vi "Main.vi"(8 "error in":errorcluster, 11 "DataSave Worker in":refnum<class "DataSave Worker.lvclass">) -> (0 "error out":errorcluster, 3 "DataSave Worker out":refnum<class "DataSave Worker.lvclass">)   [LabVIEW 2020, in "DataSave Worker.lvclass"]
doc: "The <b>Queued Message Handler</b> of the Worker that owns this VI."
uses:
  DataSave Worker.lvclass
  Initialization Data.ctl
  Response Cases.ctl
  DataSave Worker.lvclass/DataSave Worker.ctl
  rqp_Send Data.ctl
  <vilib>/Utility/file.llb/Write Delimited Spreadsheet (string).vi
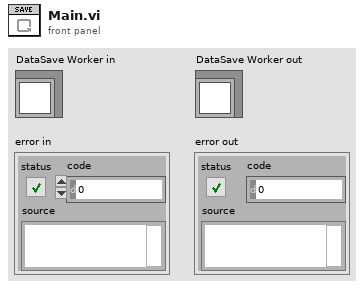
[diagram p1: front panel]
types:
  T1 = typedef "DataSave Worker.lvclass/Initialization Data.ctl" = cluster{"Response Cases":T2}
  T2 = typedef "DataSave Worker.lvclass/Response Cases.ctl" = cluster{"Placeholder - Can be deleted":string}
  T3 = typedef "DataSave Worker.lvclass/rqp_Send Data.ctl" = cluster{"Data":dbl}
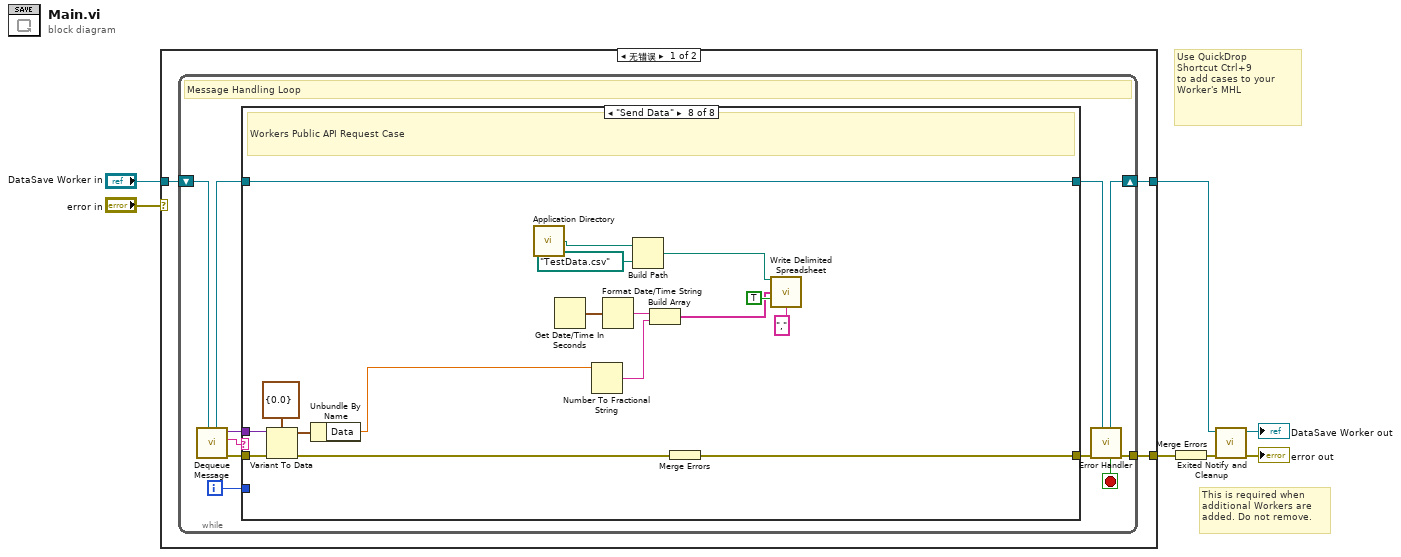
[diagram p0: block diagram]
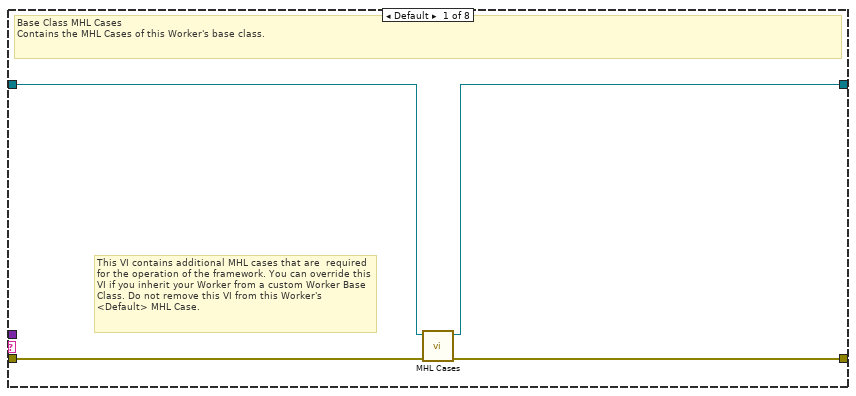
[diagram p2: hidden frame]
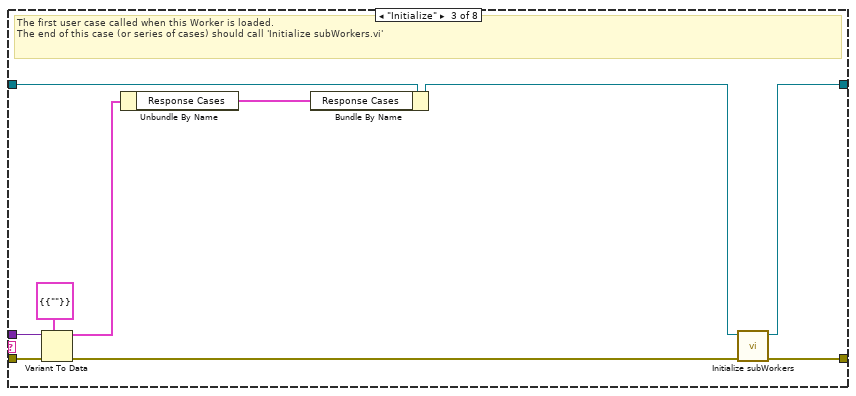
[diagram p4: hidden frame]
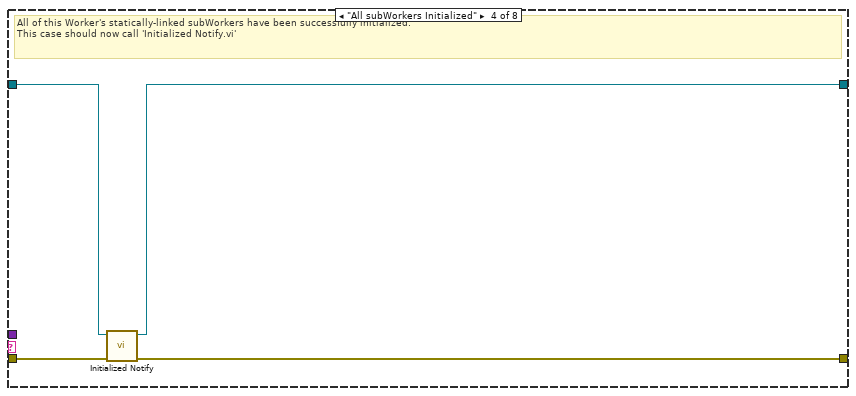
[diagram p5: hidden frame]
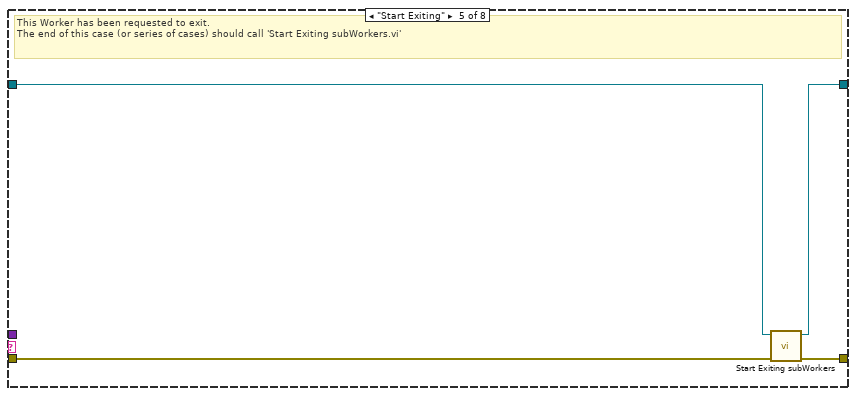
[diagram p6: hidden frame]
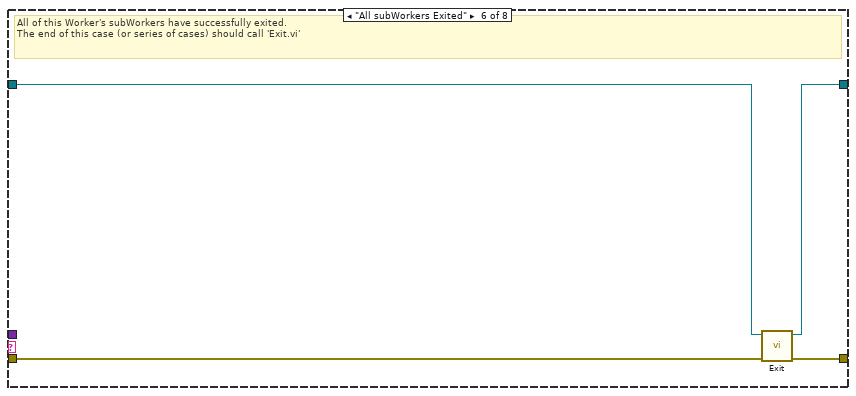
[diagram p7: hidden frame]
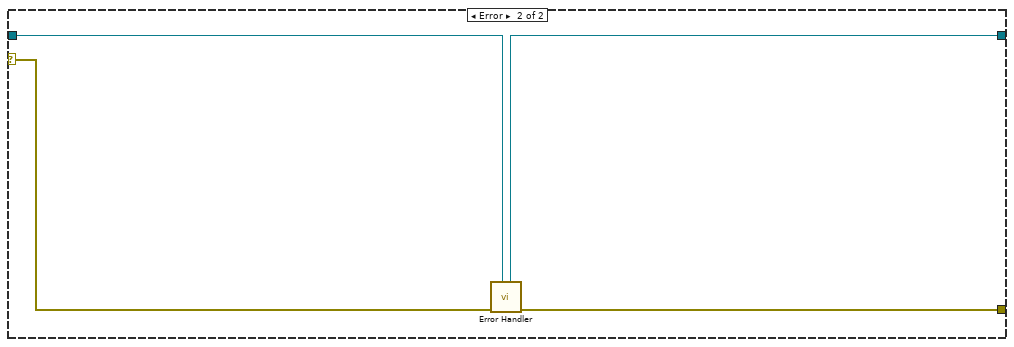
[diagram p9: hidden frame]
diagram:
  # "Use QuickDrop\nShortcut Ctrl+9\nto add cases to your\nWorker's MHL"
  # "This is required when additional Workers are added. Do not remove."
  n1 = case shown="无错误" "error in" {
    tunnel: "DataSave Worker in" -> [w8 w70]
    tunnel: [w10 w71] -> w6
    tunnel: [w9 w69] -> w7
    selector: "error in" -> [_ w72]
    frame No Error {
      n2 = while {
        shift-right: [w19] -> w9
        shift-left: w8 -> [w21]
        tunnel: [w20] -> w10
        i -> [w12]
        stop <- w13 stop-if-true
        # "Message Handling Loop"
        n3 = call-dynamic "Dequeue Message.vi"("Worker"=w21) -> ("error out"=w18:errorcluster, "Case out"=w14:string, "Data out"=w11:variant, "Worker out"=w16:refnum<class "DataSave Worker.lvclass">)  [unwired: 6 in, 1 out]
        n4 = case "Worker MHL Case Structure (DO NOT CHANGE LABEL NAME)" shown="\"Send Data\"" w14 {
          tunnel: w18 -> [w25 w26 w35 w41 w42 w49 w51 w67]
          tunnel: [w24 w26 w37 w40 w45 w48 w51 w62] -> w17
          tunnel: w16 -> [w23 w27 w34 w39 w43 w47 w50 w68]
          tunnel: [w22 w27 w36 w38 w44 w46 w50 w68] -> w15
          tunnel: w12 -> [_ _ _ _ _ _ _ _]
          tunnel: w11 -> [_ _ w32 _ _ _ _ w64]
          frame Default {
            # "This VI contains additional MHL cases that are  required for the operation of the framework. You can override this VI if you inherit your Worker from a custom Worker Base Class. Do not remove this VI from this Worker's <Default> MHL Case."
            # "Base Class MHL Cases\nContains the MHL Cases of this Worker's base class."
            n5 = call-dynamic "MHL Cases.vi"("error in"=w25, "Worker in"=w23) -> ("error out"=w24:errorcluster, "Worker out"=w22:refnum<class "DataSave Worker.lvclass">)  [unwired: 8 in]
          }
          frame "------------ FRAMEWORK CASES -----------" {
            # "Start of Workers Framework Cases"
          }
          frame "Initialize" {
            # "The first user case called when this Worker is loaded.\nThe end of this case (or series of cases) should call 'Initialize subWorkers.vi'"
            n6 = Variant To Data(error in=w35, type=T1 {"Response Cases"={"Placeholder - Can be deleted"=""}} ("Cluster"), Variant=w32) -> (data=w30:T1, error out=w33:errorcluster)
            n7 = Unbundle By Name(w30) -> ("Response Cases"=w29:T2)
            n8 = Bundle By Name(cluster=w34, "Response Cases"=w29) -> (w31:refnum<class "DataSave Worker.lvclass">)
            n9 = call-dynamic "Initialize subWorkers.vi"("error in"=w33, "Worker"=w31) -> ("error out"=w37:errorcluster, "dup Worker out"=w36:refnum<class "DataSave Worker.lvclass">)  [unwired: 8 in]
          }
          frame "All subWorkers Initialized" {
            # "All of this Worker's statically-linked subWorkers have been successfully initialized.\nThis case should now call 'Initialized Notify.vi'"
            n10 = call-dynamic "Initialized Notify.vi"("error in"=w41, "Worker"=w39) -> ("error out"=w40:errorcluster, "dup Worker out"=w38:refnum<class "DataSave Worker.lvclass">)  [unwired: 8 in]
          }
          frame "Start Exiting" {
            # "This Worker has been requested to exit. \nThe end of this case (or series of cases) should call 'Start Exiting subWorkers.vi'"
            n11 = call-dynamic "Start Exiting subWorkers.vi"("error_in"=w42, "Worker"=w43) -> ("error out"=w45:errorcluster, "dup Worker out"=w44:refnum<class "DataSave Worker.lvclass">)  [unwired: 8 in]
          }
          frame "All subWorkers Exited" {
            # "All of this Worker's subWorkers have successfully exited. \nThe end of this case (or series of cases) should call 'Exit.vi'"
            n12 = call-dynamic "Exit.vi"("error_in"=w49, "Worker"=w47) -> ("error out"=w48:errorcluster, "dup Worker out"=w46:refnum<class "DataSave Worker.lvclass">)  [unwired: 8 in]
          }
          frame "------------- PUBLIC API CASES -------------" {
            # "Start of Workers Public API Cases"
          }
          frame "Send Data" {
            # "Workers Public API Request Case"
            n13 = Variant To Data(error in=w67, type=T3 {"Data"=0.0} ("Data"), Variant=w64) -> (data=w63:T3, error out=w66:errorcluster)
            n14 = Unbundle By Name(w63) -> ("Data"=w52:dbl)
            n15 = call <vilib>:"Application Directory.vi"() -> ("Application Directory"=w57:path)
            n16 = Get Date/Time In Seconds() -> (seconds since 1Jan1904=w60:timestamp)
            n17 = Number To Fractional String(number=w52) -> (F-format string=w58:string)  [unwired: 3 in]
            n18 = Format Date/Time String(seconds (now)=w60) -> (date/time string=w59:string)  [unwired: 2 in]
            n19 = Build Path(base path=w57, name or relative path=path "TestData.csv" ("名称或相对路径")) -> (appended path=w56:path)
            n20 = Build Array(w59, w58) -> (w55:string[])
            n21 = Merge Errors(w66) -> (w62:errorcluster)
            n22 = call-poly <vilib>:"Write Delimited Spreadsheet.vi"("file path (dialog if empty)"=w56, "1D data"=w55, "append to file? (new file:F)"=TRUE, "delimiter (\\t)"="," ("delimiter (\\t)")) -> ()  [unwired: 10 in, 2 out]
          }
        }
        n23 = call-dynamic "Error Handler.vi"("Worker"=w15, "error_in"=w17) -> ("error out"=w20:errorcluster, "Stop Loop"=w13:bool, "Worker out"=w19:refnum<class "DataSave Worker.lvclass">)  [unwired: 7 in]
      }
    }
    frame Error {
      n24 = call-dynamic "Error Handler.vi"("Worker"=w70, "error_in"=w72) -> ("error out"=w71:errorcluster, "Worker out"=w69:refnum<class "DataSave Worker.lvclass">)  [unwired: 7 in, 1 out]
    }
  }
  n25 = Merge Errors(w6) -> (w3:errorcluster)
  n26 = call-dynamic "Exited Notify and Cleanup.vi"("error_in"=w3, "Worker"=w7) -> ("error out"=→"error out":errorcluster, "dup Worker out"=→"DataSave Worker out":refnum<class "DataSave Worker.lvclass">)  [unwired: 8 in]
